vi "Port Checking Error String.vi"(2 "Ch Index":i32, 3 "Port":string, 4 "Available Ports":string[](array[string])) -> (0 "error out":errorcluster)   [LabVIEW 2020]
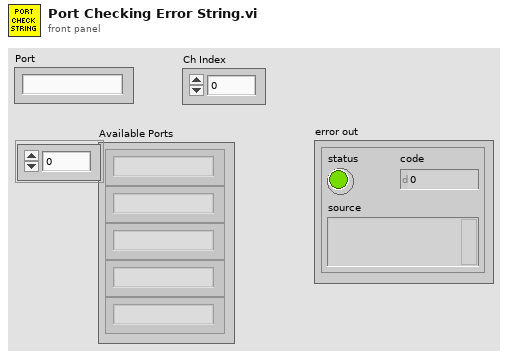
[diagram p1: front panel]
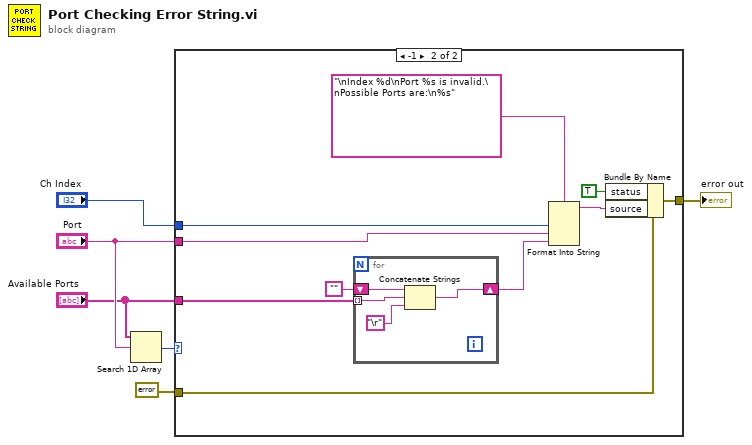
[diagram p0: block diagram]
diagram:
  n1 = Search 1D Array(1D array="Available Ports", element="Port") -> (index of element=w4:i32)  [unwired: 1 in]
  n2 = case shown="-1" w4 {
    tunnel: "Ch Index" -> [_ w13]
    tunnel: "Port" -> [_ w17]
    tunnel: "Available Ports" -> [_ w15]
    tunnel: [w7 w11] -> w1
    tunnel: errorcluster {"status"=FALSE, "code"=0, "source"=""} ("error out") -> [w7 w12]
    frame Default {
    }
    frame -1 {
      n3 = for {
        shift-right: [w18] -> w14
        shift-left: "" -> [w21]
        tunnel: w15 -> [w20] mode=indexing
        n4 = Concatenate Strings(w21, w20, "\r") -> (w18:string)
      }
      n5 = Format Into String(format string="\nIndex %d\nPort %s is invalid.\nPossible Ports are:\n%s", w13, w17, w14) -> (resulting string=w9:string)  [unwired: 2 in, 1 out]
      n6 = Bundle By Name(cluster=w12, "status"=TRUE, "source"=w9) -> (w11:errorcluster)
    }
  }
  "error out" <- w1
